vi "GEOM_ParseDiscard.vi"(9 "discard args":string, 10 "amplifiers":T1[](array[typedef]) {"fliped" items=["none", "horizontal", "vertical"]; "type" items=["LL", "LR", "UL", "UR"]}) -> (2 "amplifiers out":T1[](array[typedef]) {"fliped" items=["none", "horizontal", "vertical"]; "type" items=["LL", "LR", "UL", "UR"]})   [LabVIEW 2016]
uses:
  GEOM_Amplifier.ctl
  GEOM_AmpType.ctl
  GEOM_ROI.ctl
  GEOM_Coords.ctl
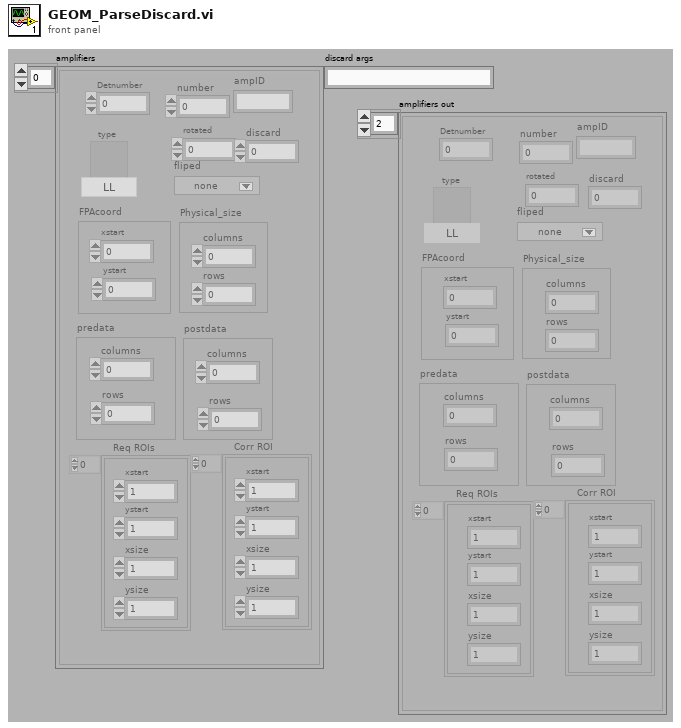
[diagram p1: front panel]
types:
  T1 = typedef "GEOM_Amplifier.ctl" = cluster{"number":i32, "type":T2, "rotated":i16, "fliped":u16, "FPAcoord":cluster{"xstart":i32, "ystart":i32}, "Physical_size":cluster{"columns":i32, "rows":i32}, "predata":cluster{"columns":i32, "rows":i32}, "postdata":cluster{"columns":i32, "rows":i32}, "Req ROIs":T3, "Corr ROI":T3, "Detnumber":i32, "ampID":string, "discard":i32}
  T2 = typedef "GEOM_AmpType.ctl" = u16
  T3 = typedef "GEOM_ROI.ctl" = T4[]
  T4 = typedef "GEOM_Coords.ctl" = cluster{"xstart":u32, "ystart":u32, "xsize":u32, "ysize":u32}
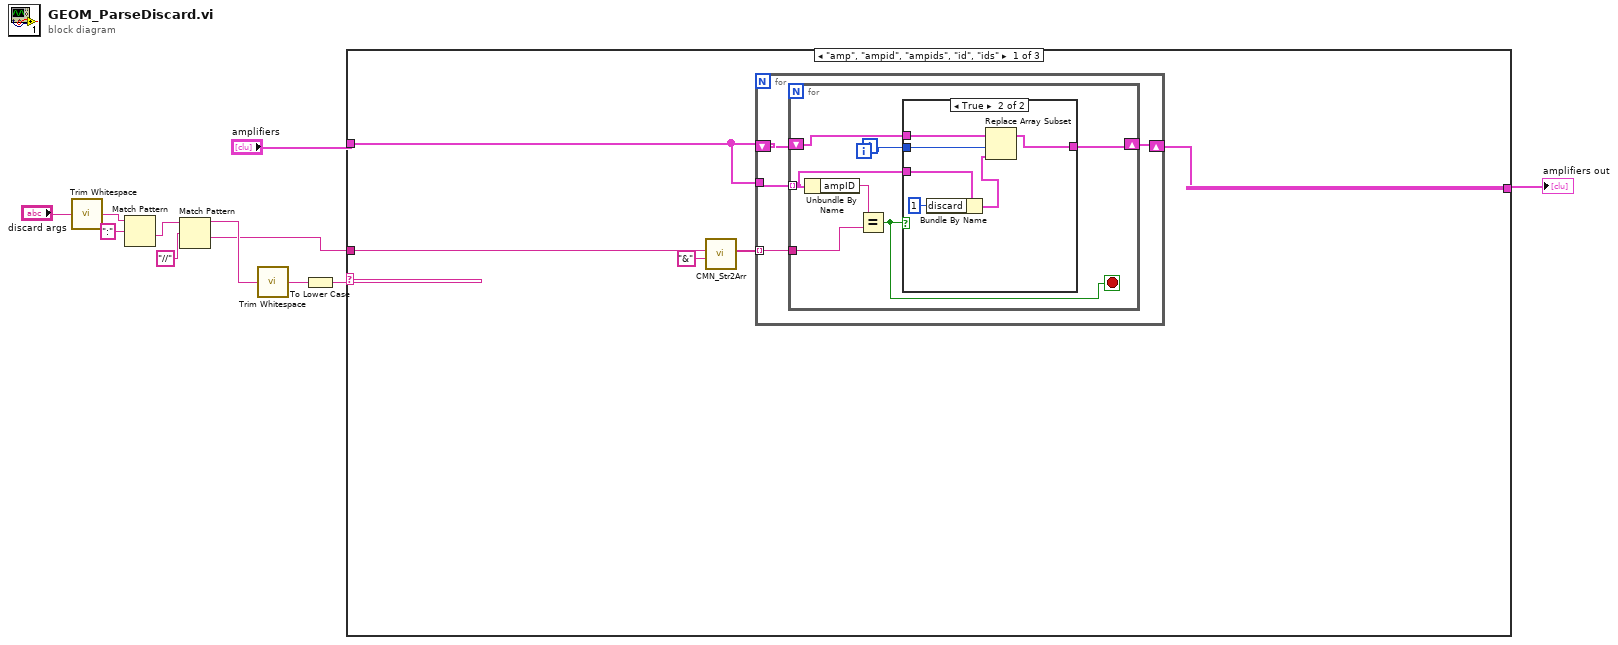
[diagram p0: block diagram]
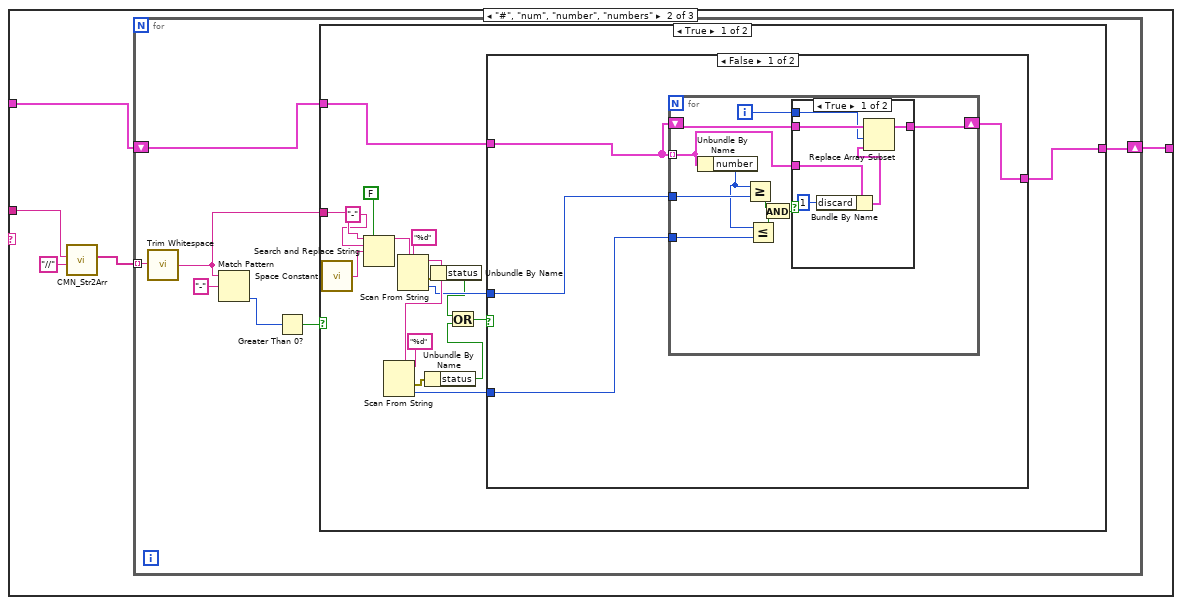
[diagram p3: hidden frame]
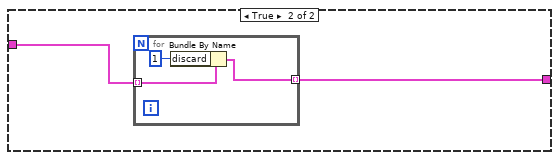
[diagram p5: hidden frame]
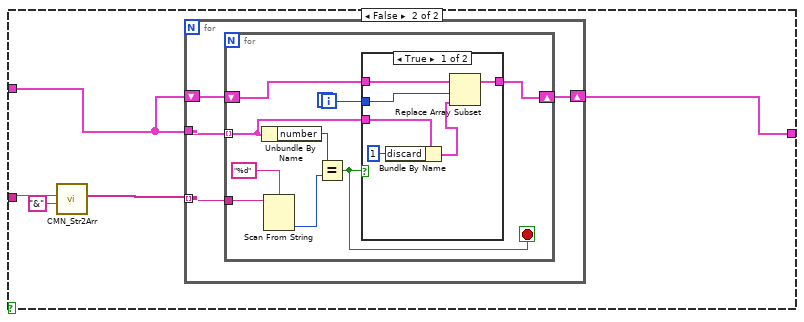
[diagram p6: hidden frame]
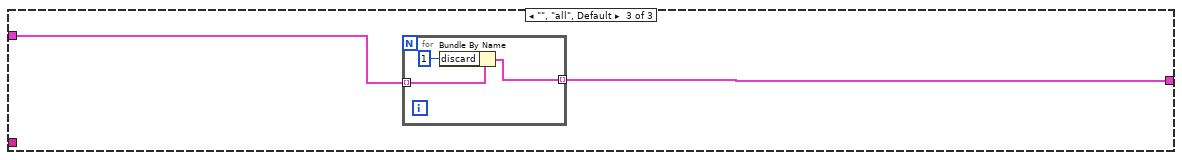
[diagram p8: hidden frame]
diagram:
  n1 = call <vilib>:"Trim Whitespace.vi"("string"="discard args") -> ("trimmed string"=w7:string)  [unwired: 1 in]
  n2 = Match Pattern(string=w7, regular expression=":") -> (after substring=w5:string)  [unwired: 4 out]
  n3 = Match Pattern(string=w5, regular expression="//") -> (before substring=w3:string, after substring=w1:string)  [unwired: 3 out]
  n4 = call <vilib>:"Trim Whitespace.vi"("string"=w3) -> ("trimmed string"=w2:string)  [unwired: 1 in]
  n5 = To Lower Case(string=w2) -> (all lower case string=w8:string)
  n6 = case shown="\"amp\", \"ampid\", \"ampids\", \"id\", \"ids\"" w8 {
    tunnel: "amplifiers" -> [w13 w35 w116]
    tunnel: [w12 w36 w115] -> w9
    tunnel: w1 -> [w16 w39 _]
    frame "amp", "ampid", "ampids", "id", "ids" {
      n7 = call "CMN_Str2Arr.vi"("separator"="&", "string in"=w16) -> ("Array out"=w14:string[])  [unwired: 2 in, 7 out]
      n8 = for {
        tunnel: w14 -> [w20] mode=indexing
        tunnel: w13 -> [w19]
        shift-right: [w17] -> w12
        shift-left: w13 -> [w18]
        n9 = for {
          tunnel: w20 -> [w26]
          tunnel: w19 -> [w25] mode=indexing
          shift-right: [w24] -> w17
          shift-left: w18 -> [w23]
          i -> [w21]
          stop <- w22 stop-if-true
          n10 = Unbundle By Name(w25) -> ("ampID"=w27:string)
          n11 = Equal?(x=w27, y=w26) -> (x = y?=w22:bool)
          n12 = case shown="True" w22 {
            tunnel: w25 -> [_ w34]
            tunnel: w23 -> [w28 w32]
            tunnel: [w28 w30] -> w24
            tunnel: w21 -> [_ w29]
            frame False {
            }
            frame True {
              n13 = Bundle By Name(cluster=w34, "discard"=1) -> (w31:T1)
              n14 = Replace Array Subset(array=w32, new element=w31, index=w29) -> (w30:T1[])
            }
          }
        }
      }
    }
    frame "#", "num", "number", "numbers" {
      n15 = call "CMN_Str2Arr.vi"("separator"="//", "string in"=w39) -> ("Array out"=w37:string[])  [unwired: 2 in, 7 out]
      n16 = for {
        tunnel: w37 -> [w43] mode=indexing
        shift-right: [w41] -> w36
        shift-left: w35 -> [w40]
        n17 = call <vilib>:"Trim Whitespace.vi"("string"=w43) -> ("trimmed string"=w42:string)  [unwired: 1 in]
        n18 = Match Pattern(string=w42, regular expression="-") -> (offset past match=w45:i32)  [unwired: 4 out]
        n19 = Greater Than 0?(x=w45) -> (x > 0?=w44:bool)
        n20 = case shown="True" w44 {
          tunnel: w40 -> [w63 w93]
          tunnel: [w62 w90] -> w41
          tunnel: w42 -> [w61 w91]
          frame True {
            n21 = call <vilib>:"Space Constant.vi"() -> ("String"=w59:string)
            n22 = Search and Replace String(replace all?=FALSE ("replace all? (F)"), input string=w61, search string="-" ("substring (\"\")"), replace string=w59) -> (result string=w58:string)  [unwired: 1 in, 6 out]
            n23 = Scan From String(format string="%d", input string=w58) -> (remaining string=w57:string, error out=w53:errorcluster, output 1=w49:i32)  [unwired: 2 in, 2 out]
            n24 = Scan From String(format string="%d", input string=w57) -> (error out=w52:errorcluster, output 1=w48:i32)  [unwired: 2 in, 3 out]
            n25 = Unbundle By Name(w52) -> ("status"=w51:bool)
            n26 = Unbundle By Name(w53) -> ("status"=w47:bool)
            n27 = Or(x=w47, y=w51) -> (x .or. y?=w50:bool)
            n28 = case shown="False" w50 {
              tunnel: w63 -> [w67 w86]
              tunnel: [w66 w85] -> w62
              tunnel: w49 -> [w65 _]
              tunnel: w48 -> [w64 _]
              frame False {
                n29 = for {
                  tunnel: w67 -> [w74] mode=indexing
                  tunnel: w65 -> [w77]
                  tunnel: w64 -> [w75]
                  shift-right: [w69] -> w66
                  shift-left: w67 -> [w70]
                  i -> [w68]
                  n30 = Unbundle By Name(w74) -> ("number"=w76:i32)
                  n31 = Greater Or Equal?(x=w76, y=w77) -> (x >= y?=w73:bool)
                  n32 = Less Or Equal?(x=w76, y=w75) -> (x <= y?=w72:bool)
                  n33 = And(x=w73, y=w72) -> (x .and. y?=w71:bool)
                  n34 = case shown="True" w71 {
                    tunnel: w74 -> [w83 _]
                    tunnel: w70 -> [w81 w84]
                    tunnel: [w79 w84] -> w69
                    tunnel: w68 -> [w78 _]
                    frame True {
                      n35 = Bundle By Name(cluster=w83, "discard"=1) -> (w80:T1)
                      n36 = Replace Array Subset(array=w81, new element=w80, index=w78) -> (w79:T1[])
                    }
                    frame False {
                    }
                  }
                }
              }
              frame True {
                n37 = for {
                  tunnel: [w88] -> w85 mode=indexing
                  tunnel: w86 -> [w87] mode=indexing
                  n38 = Bundle By Name(cluster=w87, "discard"=1) -> (w88:T1)
                }
              }
            }
          }
          frame False {
            n39 = call "CMN_Str2Arr.vi"("separator"="&", "string in"=w91) -> ("Array out"=w92:string[])  [unwired: 2 in, 7 out]
            n40 = for {
              tunnel: w92 -> [w97] mode=indexing
              tunnel: w93 -> [w98]
              shift-right: [w95] -> w90
              shift-left: w93 -> [w96]
              n41 = for {
                tunnel: w98 -> [w106] mode=indexing
                tunnel: w97 -> [w105]
                shift-right: [w101] -> w95
                shift-left: w96 -> [w102]
                i -> [w99]
                stop <- w100 stop-if-true
                n42 = Unbundle By Name(w106) -> ("number"=w107:i32)
                n43 = Scan From String(format string="%d", input string=w105) -> (output 1=w103:i32)  [unwired: 2 in, 4 out]
                n44 = Equal?(x=w107, y=w103) -> (x = y?=w100:bool)
                n45 = case shown="True" w100 {
                  tunnel: w106 -> [w113 _]
                  tunnel: w102 -> [w110 w114]
                  tunnel: [w109 w114] -> w101
                  tunnel: w99 -> [w108 _]
                  frame True {
                    n46 = Bundle By Name(cluster=w113, "discard"=1) -> (w111:T1)
                    n47 = Replace Array Subset(array=w110, new element=w111, index=w108) -> (w109:T1[])
                  }
                  frame False {
                  }
                }
              }
            }
          }
        }
      }
    }
    frame "", "all", Default {
      n48 = for {
        tunnel: [w118] -> w115 mode=indexing
        tunnel: w116 -> [w117] mode=indexing
        n49 = Bundle By Name(cluster=w117, "discard"=1) -> (w118:T1)
      }
    }
  }
  "amplifiers out" <- w9
